vi "TCP-IMG-Sender.vi"() -> ()   [LabVIEW 2019]
panel:
  in  "Stop":bool
  out "Image":T1(plugin-control)
  # "TCP Image Sender"
  # "Instructions:\n1.  Run this VI.\n2.  Run \"TCP-IMG-Receiver\".\n3. See the images transfered via TCP."
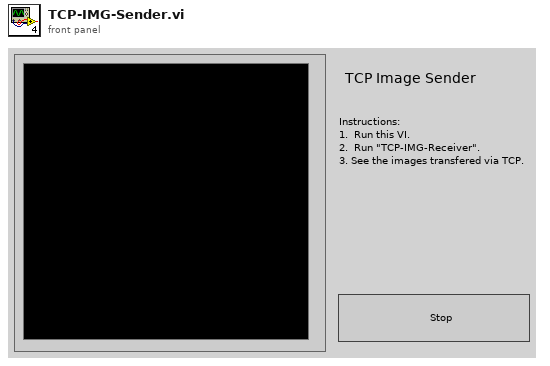
[diagram p1: front panel]
types:
  T1 = typedef "IMAQ Image.ctl" = refnum<image>
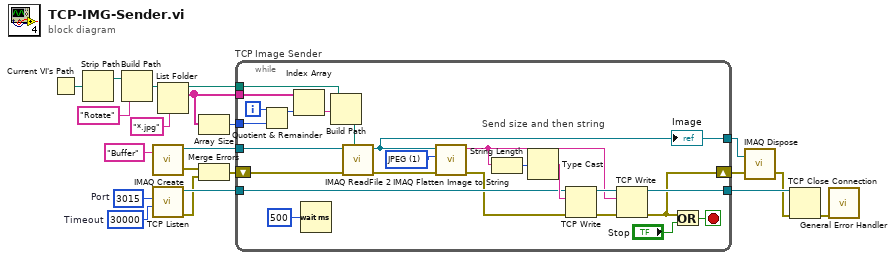
[diagram p0: block diagram]
diagram:
  w20 = 30000  # Timeout
  w19 = u16 3015  # Port
  n1 = Current VI's Path() -> (path=w11:path)
  n2 = Strip Path(path=w11) -> (stripped path=w10:path)  [unwired: 1 out]
  n3 = Build Path(base path=w10, name or relative path="Rotate") -> (appended path=w8:path)
  n4 = call "IMAQ Create"("Image Name"="Buffer") -> ("New Image"=w21:T1, "error out"=w2:errorcluster)  [unwired: 4 in]
  n5 = call <vilib>:"TCP Listen.vi"("timeout ms (wait forever: -1)"=w20, "port"=w19) -> ("error out"=w17:errorcluster, "connection ID"=w18:refnum<k5>)  [unwired: 5 in, 3 out]
  n6 = List Folder(path=w8, pattern="*.jpg") -> (path out=w6:path, filenames=w4:string[])  [unwired: 2 in, 2 out]
  n7 = Array Size(array=w4) -> (size(s)=w5:i32)
  n8 = Merge Errors(w2, w17) -> (w16:errorcluster)
  n9 = while "TCP Image Sender" {
    tunnel: w21 -> [w25]
    tunnel: w18 -> [w41]
    shift-right: [w26] -> w13
    shift-left: w16 -> [w28]
    tunnel: [w40] -> w15
    tunnel: [w24] -> w14
    tunnel: w6 -> [w34]
    tunnel: w5 -> [w31]
    tunnel: w4 -> [w30]
    i -> [w32]
    stop <- w36 stop-if-true
    w39 = 1 items=["None", "JPEG", "PACKED BINARY"] ("Compression (None)")
    # "Send size and then string"
    n10 = Quotient & Remainder(x=w32, y=w31) -> (x-y*floor(x/y)=w35:i32)  [unwired: 1 out]
    n11 = Index Array(array=w30, index=w35) -> (element=w33:string)
    n12 = Wait (ms)(milliseconds to wait=u32 500) -> ()  [unwired: 1 out]
    n13 = Build Path(base path=w34, name or relative path=w33) -> (appended path=w29:path)
    n14 = call "IMAQ ReadFile 2"("File Path"=w29, "error in (no error)"=w28, "Image"=w25) -> ("error out"=w27:errorcluster, "Image Out"=w24:T1)  [unwired: 4 in, 3 out]
    "Image" <- w24
    n15 = call "IMAQ Flatten Image to String"("error in (no error)"=w27, "Compression (None)"=w39, "Image"=w24) -> ("error out"=w37:errorcluster, "Data String"=w38:string)  [unwired: 7 in]
    n16 = String Length(string=w38) -> (length=w42:i32)
    n17 = Type Cast(x=w42) -> (*(type *) &x=w43:string)  [unwired: 1 in]
    n18 = TCP Write(connection ID=w41, data in=w43, error in (no error)=w37) -> (connection ID out=w44:refnum<k5>, error out=w45:errorcluster)  [unwired: 1 in, 1 out]
    n19 = TCP Write(connection ID=w44, data in=w38, error in (no error)=w45) -> (connection ID out=w40:refnum<k5>, error out=w26:errorcluster)  [unwired: 1 in, 1 out]
    n20 = Or(x=w26, y="Stop") -> (x .or. y?=w36:bool)
  }
  n21 = call "IMAQ Dispose"("Image"=w14, "error in (no error)"=w13) -> ("error out"=w1:errorcluster)  [unwired: 4 in]
  n22 = TCP Close Connection(connection ID=w15, error in (no error)=w1) -> (error out=w12:errorcluster)  [unwired: 1 in, 1 out]
  n23 = call <vilib>:"General Error Handler.vi"("error in (no error)"=w12) -> ()  [unwired: 10 in, 5 out]
